vi "Reading_Proc.vi"(8 "y":i32, 9 "x":i32, 10 "task/channels in 2":refnum<k21>, 11 "task/channels in":refnum<k21>) -> (1 "data":bool, 2 "task out 2":refnum<k21>, 3 "task out":refnum<k21>)   [LabVIEW 2018]
uses:
  <vilib>/DAQmx/read.llb/DAQmx Read (Digital Bool 1Line 1Point).vi
  <vilib>/DAQmx/write.llb/DAQmx Write (Digital Bool 1Line 1Point).vi
  <vilib>/DAQmx/miscellaneous.llb/DAQmx Fill In Error Info.vi
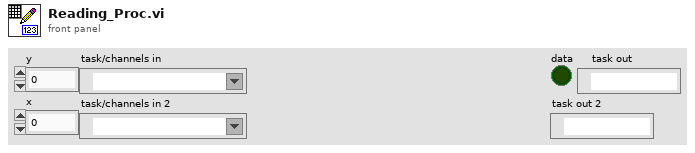
[diagram p1: front panel]
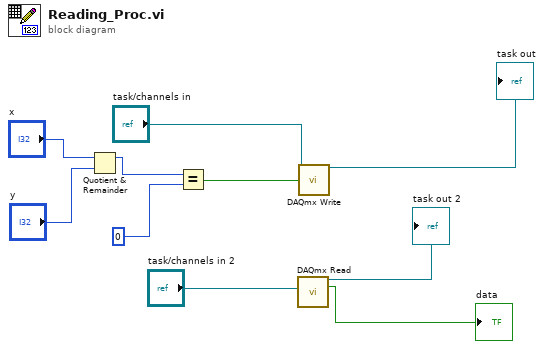
[diagram p0: block diagram]
diagram:
  n1 = Quotient & Remainder(x="x", y="y") -> (x-y*floor(x/y)=w8:i32)  [unwired: 1 out]
  n2 = Equal?(x=w8, y=0) -> (x = y?=w6:bool)
  n3 = call-poly <vilib>:"DAQmx Read.vi"("task/channels in"="task/channels in 2") -> ("task out"=→"task out 2":refnum<k21>, "data"=→"data":bool)  [unwired: 12 in, 1 out]
  n4 = call-poly <vilib>:"DAQmx Write.vi"("task/channels in"="task/channels in", "data"=w6) -> ("task out"=→"task out":refnum<k21>)  [unwired: 11 in, 2 out]
